vi "setScriptPath.vi"(8 "error in (no error)":errorcluster, 10 "dpScriptPath":path, 11 "Point.lvclass in":refnum<class "Point.lvclass">) -> (0 "error out":errorcluster, 3 "Point.lvclass out":refnum<class "Point.lvclass">)   [LabVIEW 2009, in "Tools.lvlib" / "Sequencing.lvlib" / "Point.lvclass"]
uses:
  Point.lvclass
  Point.lvclass/Point.ctl
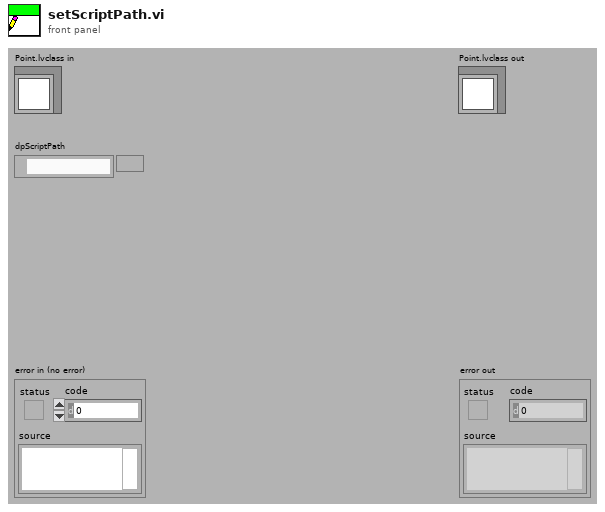
[diagram p1: front panel]
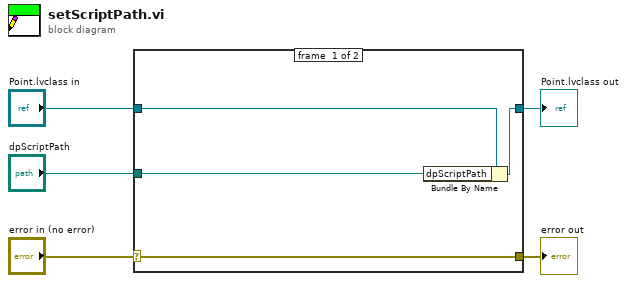
[diagram p0: block diagram]
diagram:
  n1 = case shown="No Error" "error in (no error)" {
    selector: "error in (no error)" -> [w9 w10]
    tunnel: [w9 w10] -> w4
    tunnel: [w7 w11] -> w2
    tunnel: "Point.lvclass in" -> [w8 w11]
    tunnel: "dpScriptPath" -> [w6 _]
    frame #0 {
      n2 = Bundle By Name(cluster=w8, "dpScriptPath"=w6) -> (w7:refnum<class "Point.lvclass">)
    }
    frame #1 {
    }
  }
  "error out" <- w4
  "Point.lvclass out" <- w2
